vi "sum.vi"(0 "X range output":u16[](array[numeric]), 5 "Y range Max output":u16[](array[numeric]), 7 "Y range Min output":u16[](array[numeric]), 11 "error in (no error)":errorcluster, 12 "Energy 2d gate out":T1, 14 "Peak height  in":u16[][](array[numeric])) -> (1 "Peak height out":u16[][](array[numeric]), 3 "sum of counts out":i32, 4 "X output array":u16[](array[numeric]), 6 "Y range  output":u16[](array[numeric]), 15 "error out":errorcluster)   [LabVIEW 2016]
doc: "This vi sorts each event and determines if it lies within a 2d bound area"
uses:
  controls/energy 2d selection.ctl
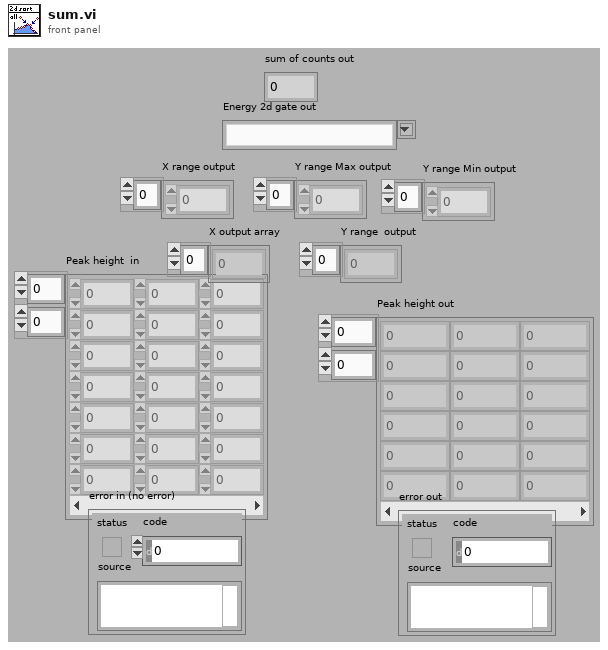
[diagram p1: front panel]
types:
  T1 = typedef "energy 2d selection.ctl" = string
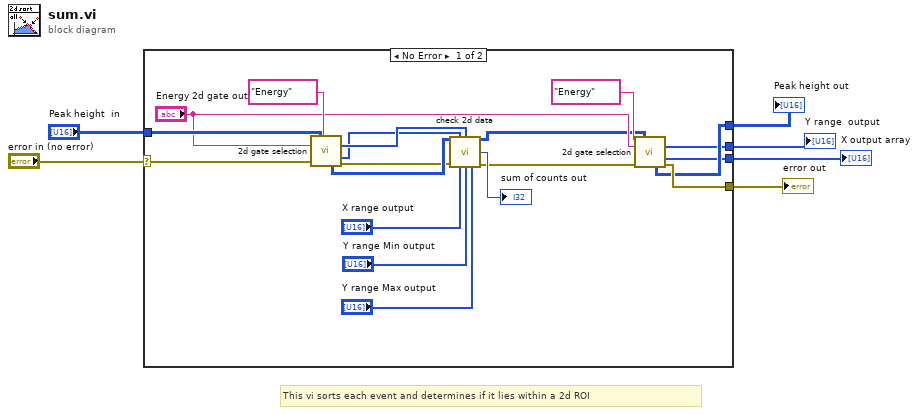
[diagram p0: block diagram]
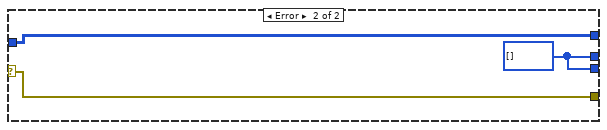
[diagram p2: hidden frame]
diagram:
  # "This vi sorts each event and determines if it lies within a 2d ROI"
  n1 = case shown="No Error" "error in (no error)" {
    selector: "error in (no error)" -> [w15 w27]
    tunnel: "Peak height  in" -> [w25 w28]
    tunnel: [w7 w26] -> w5
    tunnel: [w8 w26] -> w4
    tunnel: [w9 w28] -> w3
    tunnel: [w12 w27] -> w1
    frame No Error {
      n2 = call "2d gate selection.vi"("time or energy"="Energy", "channel 0-4 energy in"=w25, "Energy 2d gate"="Energy 2d gate out", "error in (no error)"=w15) -> ("Y output array"=w11:i32[], "X output array"=w10:i32[], "channel 0-4 energy out"=w16:u32[][], "error out (no error)"=w14:errorcluster)  [unwired: 5 in, 3 out]
      n3 = call "check 2d data.vi"("Peak height in"=w16, "X input"=w10, "Y input"=w11, "error in (no error)"=w14, "X gate input"="X range output", "gate y min"="Y range Min output", "gate y max"="Y range Max output") -> ("Peak height out"=w21:u16[][], "sum of counts out"=→"sum of counts out":u32, "error out"=w13:errorcluster)  [unwired: 5 in, 1 out]
      n4 = call "2d gate selection.vi"("time or energy"="Energy", "channel 0-4 energy in"=w21, "Energy 2d gate"="Energy 2d gate out", "error in (no error)"=w13) -> ("Y output array"=w7:i32[], "X output array"=w8:i32[], "channel 0-4 energy out"=w9:u32[][], "error out (no error)"=w12:errorcluster)  [unwired: 5 in, 3 out]
    }
    frame Error {
      w26 = u32[] [] ("Y output array")
    }
  }
  "Peak height out" <- w3
  "X output array" <- w4
  "Y range  output" <- w5
  "error out" <- w1
